vi "Router - Connect.vi"(8 "error in (no error)":errorcluster, 10 "Configuration Properties":T1, 11 "Router Data In":T4) -> (0 "error out":errorcluster, 2 "Configuration Properties Out":T1, 3 "Router Data Out":T4)   [LabVIEW 2016, in "PXImc Router.lvlib"]
uses:
  PXImc Router.lvlib
  Controls/Router - Configuration.ctl
  Controls/Node Properties.ctl
  Controls/Table Index-Size.ctl
  Controls/Router Data.ctl
  Controls/Reader Data.ctl
  Controls/Writer Data.ctl
  <vilib>/pximc/Connect (DBL).vi
  <vilib>/pximc/nipximc.lvlib
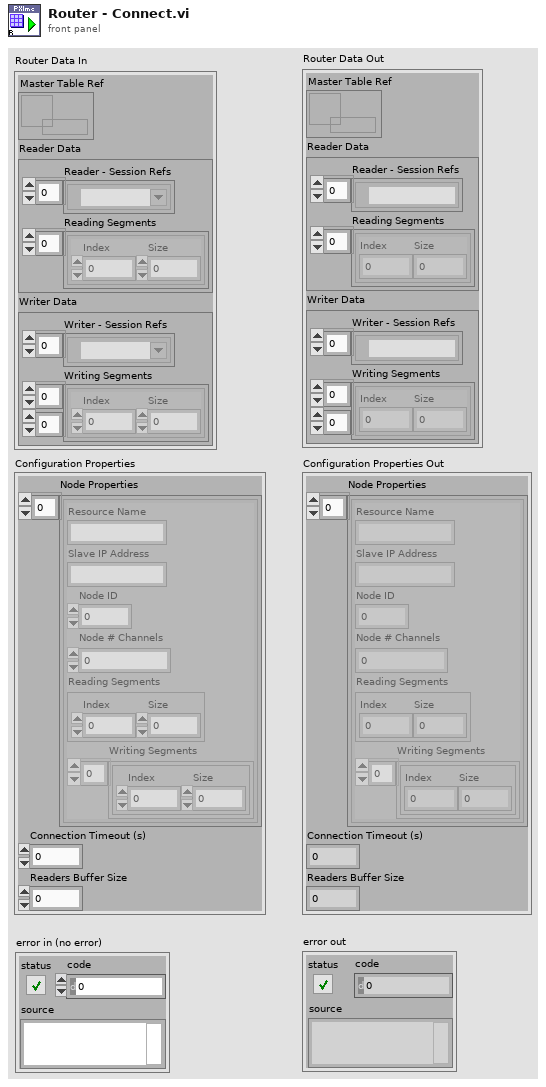
[diagram p1: front panel]
types:
  T1 = typedef "PXImc Router.lvlib/Router - Configuration.ctl" = cluster{"Node Properties":T2[], "Connection Timeout (s)":dbl, "Readers Buffer Size":u32}
  T2 = typedef "PXImc Router.lvlib/Node Properties.ctl" = cluster{"Resource Name":string, "Slave IP Address":string, "Node ID":u16, "Node # Channels":u32, "Reading Segments":T3, "Writing Segments":T3[]}
  T3 = typedef "PXImc Router.lvlib/Table Index-Size.ctl" = cluster{"Index":u32, "Size":u32}
  T4 = typedef "PXImc Router.lvlib/Router Data.ctl" = cluster{"Master Table Ref":refnum<data-value>, "Reader Data":T5, "Writer Data":T6}
  T5 = typedef "PXImc Router.lvlib/Reader Data.ctl" = cluster{"Reader - Session Refs":refnum<k21>[], "Reading Segments":T3[]}
  T6 = typedef "PXImc Router.lvlib/Writer Data.ctl" = cluster{"Writer - Session Refs":refnum<k21>[], "Writing Segments":T3[][]}
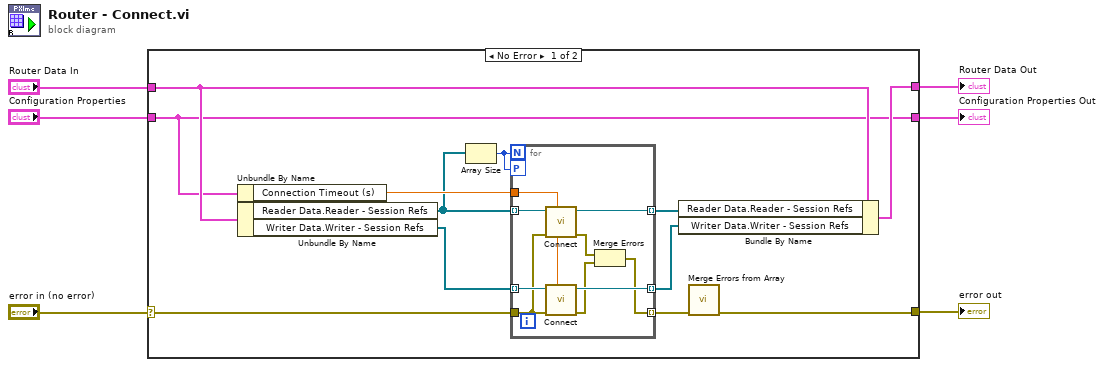
[diagram p0: block diagram]
diagram:
  n1 = case shown="No Error" "error in (no error)" {
    selector: "error in (no error)" -> [w7 w28]
    tunnel: "Configuration Properties" -> [w9 w29]
    tunnel: "Router Data In" -> [w13 w30]
    tunnel: [w11 w30] -> w4
    tunnel: [w9 w29] -> w3
    tunnel: [w8 w28] -> w1
    frame No Error {
      n2 = Unbundle By Name(w9) -> ("Connection Timeout (s)"=w16:dbl)
      n3 = Unbundle By Name(w13) -> ("Reader Data.Reader - Session Refs"=w12:refnum<k21>[], "Writer Data.Writer - Session Refs"=w17:refnum<k21>[])
      n4 = Array Size(array=w12) -> (size(s)=w18:i32)
      n5 = for {
        N: w18 -> [_]
        tunnel: [w27] -> w14 mode=indexing
        tunnel: [w26] -> w15 mode=indexing
        tunnel: w16 -> [w25]
        tunnel: w12 -> [w24] mode=indexing
        tunnel: w17 -> [w23] mode=indexing
        workers-P: w18 -> [_]
        tunnel: w7 -> [w22]
        tunnel: [w19] -> w10 mode=indexing
        n6 = call-poly <vilib>:"Connect.vi"("timeout in seconds (-1)"=w25, "error in (no error)"=w22, "session in"=w24) -> ("error out"=w21:errorcluster, "session out"=w26:refnum<k21>)  [unwired: 7 in]
        n7 = call-poly <vilib>:"Connect.vi"("timeout in seconds (-1)"=w25, "error in (no error)"=w22, "session in"=w23) -> ("error out"=w20:errorcluster, "session out"=w27:refnum<k21>)  [unwired: 7 in]
        n8 = Merge Errors(w21, w20) -> (w19:errorcluster)
      }
      n9 = Bundle By Name(cluster=w13, "Reader Data.Reader - Session Refs"=w15, "Writer Data.Writer - Session Refs"=w14) -> (w11:T4)
      n10 = call "Merge Errors from Array.vi"("Error Array In"=w10) -> ("error out"=w8:errorcluster)  [unwired: 10 in]
    }
    frame Error {
    }
  }
  "Router Data Out" <- w4
  "Configuration Properties Out" <- w3
  "error out" <- w1
